vi "Looper.vi"(9 "Num Points":dbl, 10 "Max":dbl, 11 "Min":dbl) -> (1 "Result":dbl[](array[numeric]), 2 "Result (str)":string[](array[string]))   [LabVIEW 2018]
panel:
  out "Delta":dbl
  out "Step Size":dbl
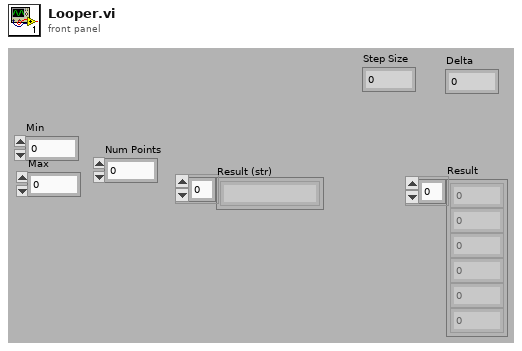
[diagram p1: front panel]
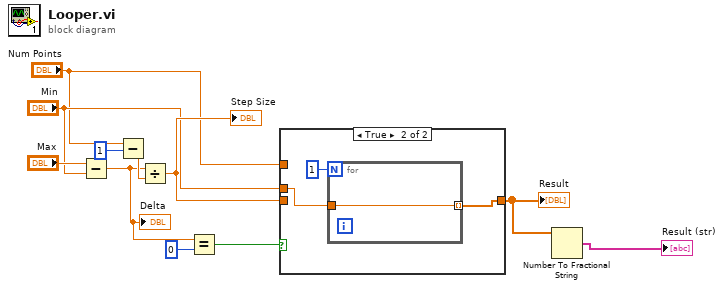
[diagram p0: block diagram]
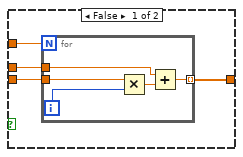
[diagram p2: hidden frame]
diagram:
  n1 = Subtract(x="Max", y="Min") -> (x-y=w5:dbl)
  "Delta" <- w5
  n2 = Subtract(x="Num Points", y=1) -> (x-y=w7:dbl)
  n3 = Divide(x=w5, y=w7) -> (x/y=w10:dbl)
  "Step Size" <- w10
  n4 = Equal?(x=w5, y=0) -> (x = y?=w3:bool)
  n5 = case shown="True" w3 {
    tunnel: w10 -> [w15 _]
    tunnel: "Min" -> [w14 w21]
    tunnel: "Num Points" -> [w13 _]
    tunnel: [w12 w23] -> w2
    frame False {
      n6 = for {
        N: w13 -> [_]
        tunnel: w14 -> [w17]
        tunnel: w15 -> [w19]
        tunnel: [w16] -> w12 mode=indexing
        i -> [w20]
        n7 = Multiply(x=w19, y=w20) -> (x*y=w18:dbl)
        n8 = Add(x=w17, y=w18) -> (x+y=w16:dbl)
      }
    }
    frame True {
      n9 = for {
        N: 1 -> [_]
        tunnel: [w24] -> w23 mode=indexing
        tunnel: w21 -> [w24]
      }
    }
  }
  "Result" <- w2
  n10 = Number To Fractional String(number=w2) -> (F-format string=→"Result (str)":string[])  [unwired: 3 in]
